vi "Scott -- strain -- sweep Init V0.vi"(11 "strain sweep control":T1={"just in case"=TRUE, "Piezo Amplifier settings"={"Gain "=69.44, "offset (V)"=69.44}, "voltage-parameters-IN"={"phase "=2.88, "amplitude (V)"=-0.7854, "offset (V)"=0.28, "time delay (sec)"=0.5, "period (sec)"=50.0, "shape"=enum."triangle"}, "Lockin Settings"=[{"Offset"=FALSE, "GPIB Address"=6}, {"Offset"=TRUE, "GPIB Address"=7}], "VISA address Agilent  IN"="", "number of iterations"=1.0, "Piezo sweep settings"={"max Piezo voltage (V) "=69.44, "min Piezo voltage (V)"=69.44, "delay (sec)"=69.44, "period (sec)"=69.44, "shape"=enum."triangle"}}) -> (0 "data array":dbl[][](array[numeric]), 1 "plots control OUT":cluster{"data string in":string, bool, bool}[](array[cluster]), 2 "total number of points":dbl=114.59, 3 "strain sweep control OUT":T1={"just in case"=TRUE, "Piezo Amplifier settings"={"Gain "=69.44, "offset (V)"=69.44}, "voltage-parameters-IN"={"phase "=2.88, "amplitude (V)"=-0.7854, "offset (V)"=0.28, "time delay (sec)"=0.5, "period (sec)"=50.0, "shape"=enum."triangle"}, "Lockin Settings"=[{"Offset"=FALSE, "GPIB Address"=6}, {"Offset"=TRUE, "GPIB Address"=7}], "VISA address Agilent  IN"="", "number of iterations"=1.0, "Piezo sweep settings"={"max Piezo voltage (V) "=69.44, "min Piezo voltage (V)"=69.44, "delay (sec)"=69.44, "period (sec)"=69.44, "shape"=enum."triangle"}})   [LabVIEW 2014]
uses:
  Scott -- strain -- strain sweep control.ctl
  FSU/ScottRiggs/Piezo2/voltage-wave-generator-parameters.ctl
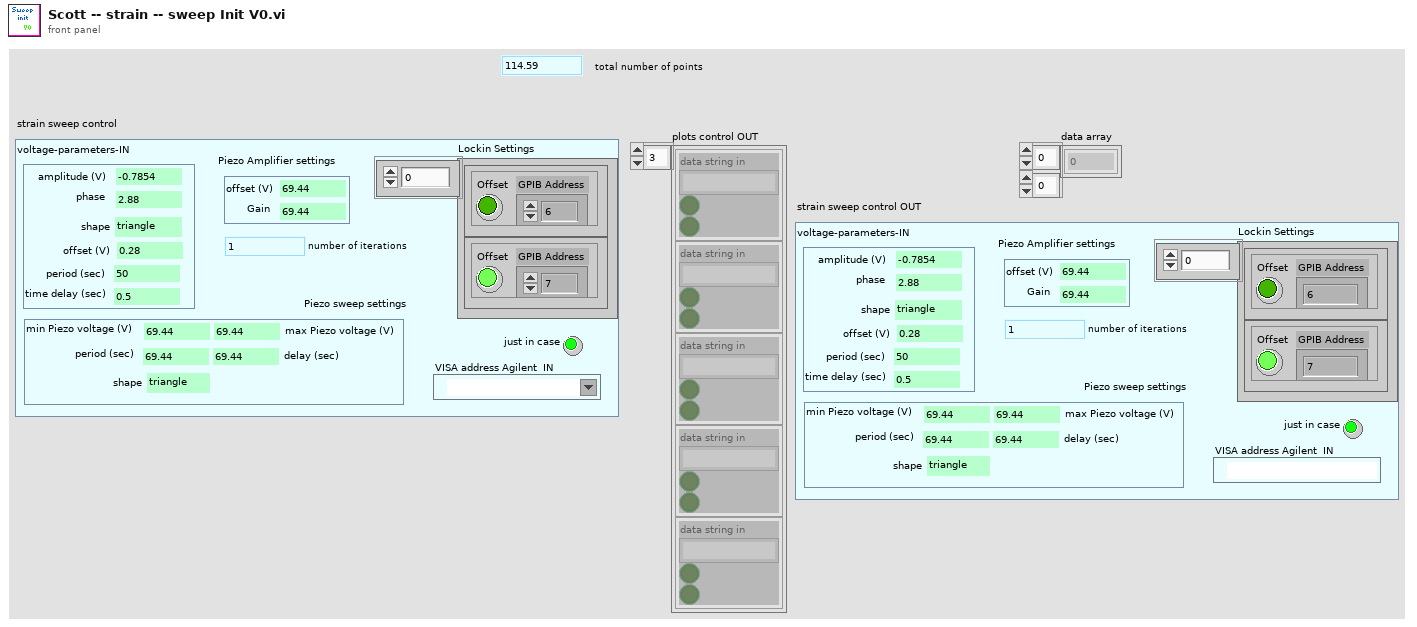
[diagram p1: front panel]
types:
  T1 = typedef "Scott -- strain -- strain sweep control.ctl" = cluster{"just in case":bool, "Piezo Amplifier settings":cluster{"Gain ":dbl, "offset (V)":dbl}, "voltage-parameters-IN":T2, "Lockin Settings":cluster{"Offset":bool, "GPIB Address":i16}[], "VISA address Agilent  IN":refnum<visa-resource-name>, "number of iterations":dbl, "Piezo sweep settings":cluster{"max Piezo voltage (V) ":dbl, "min Piezo voltage (V)":dbl, "delay (sec)":dbl, "period (sec)":dbl, "shape":enum16{"triangle", "sine", "none"}}}
  T2 = typedef "voltage-wave-generator-parameters.ctl" = cluster{"phase ":dbl, "amplitude (V)":dbl, "offset (V)":dbl, "time delay (sec)":dbl, "period (sec)":dbl, "shape":enum16{"triangle", "sine", "none"}}
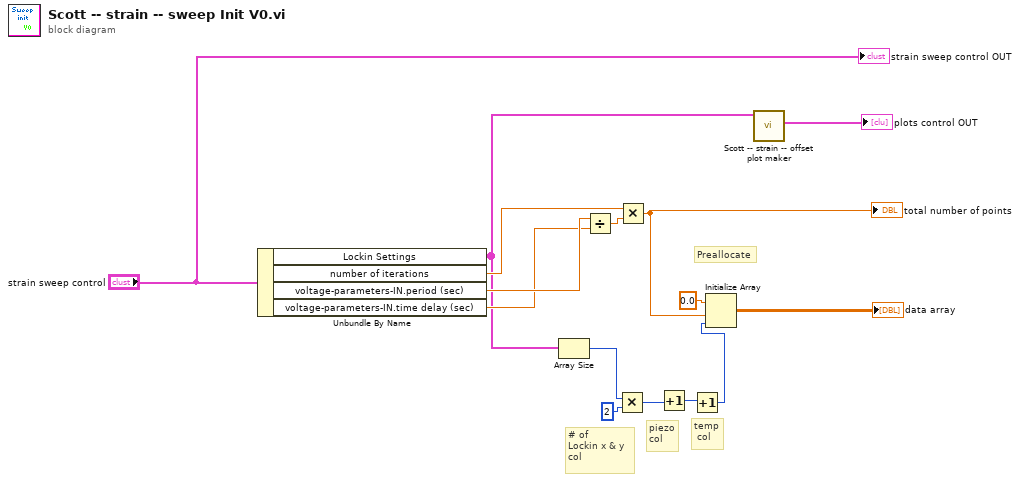
[diagram p0: block diagram]
diagram:
  # "temp\n col"
  # "piezo\ncol"
  # "# of \nLockin x & y\ncol"
  # "Preallocate"
  n1 = Unbundle By Name("strain sweep control") -> ("Lockin Settings"=w10:cluster{"Offset":bool, "GPIB Address":i16}[], "number of iterations"=w12:dbl, "voltage-parameters-IN.period (sec)"=w15:dbl, "voltage-parameters-IN.time delay (sec)"=w14:dbl)
  n2 = Array Size(array=w10) -> (size(s)=w1:i32)
  n3 = Divide(x=w15, y=w14) -> (x/y=w13:dbl)
  n4 = Multiply(x=w1, y=2) -> (x*y=w4:i32)
  n5 = Multiply(x=w12, y=w13) -> (x*y=w11:dbl)
  "total number of points" <- w11
  n6 = Increment(x=w4) -> (x+1=w3:i32)
  n7 = Increment(x=w3) -> (x+1=w2:i32)
  n8 = Initialize Array(0.0 ("element"), w11, w2) -> (→"data array":dbl[][])
  n9 = call "Scott -- strain -- offset plot maker.vi"("Lockin Settings"=w10) -> ("appended array"=→"plots control OUT":cluster{"data string in":string, bool, bool}[])  [unwired: 9 in, 1 out]
  "strain sweep control OUT" <- "strain sweep control"
